vi "Read Square Index.vi"(8 "error in (no error)":errorcluster, 11 "AndrewF in":refnum<class "AndrewF.lvclass">) -> (0 "error out":errorcluster, 2 "Square Index":i32, 3 "AndrewF out":refnum<class "AndrewF.lvclass">)   [LabVIEW 2015, in "AndrewF.lvclass"]
uses:
  AndrewF.lvclass
  AndrewF.lvclass/AndrewF.ctl
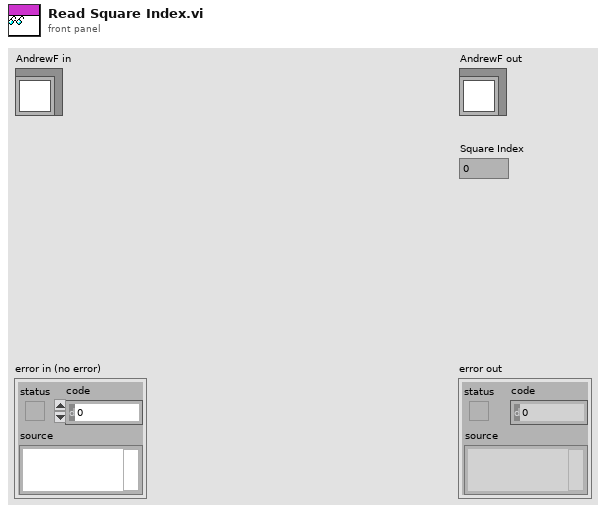
[diagram p1: front panel]
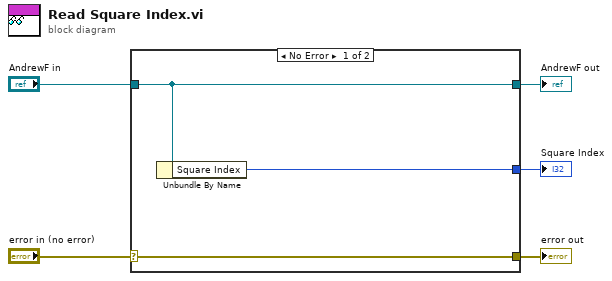
[diagram p0: block diagram]
diagram:
  n1 = case shown="No Error" "error in (no error)" {
    selector: "error in (no error)" -> [w8 w9]
    tunnel: [w8 w9] -> w4
    tunnel: [w7 w10] -> w2
    tunnel: "AndrewF in" -> [w7 w10]
    tunnel: [w6 _] -> w1
    frame No Error {
      n2 = Unbundle By Name(w7) -> ("Square Index"=w6:i32)
    }
    frame Error {
    }
  }
  "error out" <- w4
  "AndrewF out" <- w2
  "Square Index" <- w1
